vi "write initial config.vi"(8 "error in (no error)":errorcluster, 11 "Channel in":refnum<class "Channel.lvclass">) -> (0 "error out":errorcluster, 3 "Channel out":refnum<class "Channel.lvclass">)   [LabVIEW 2018, in "Channel.lvclass"]
uses:
  Channel.lvclass
  Channel.lvclass/Channel.ctl
  Simulated_CCD_Camera/Simulated Camera.lvclass
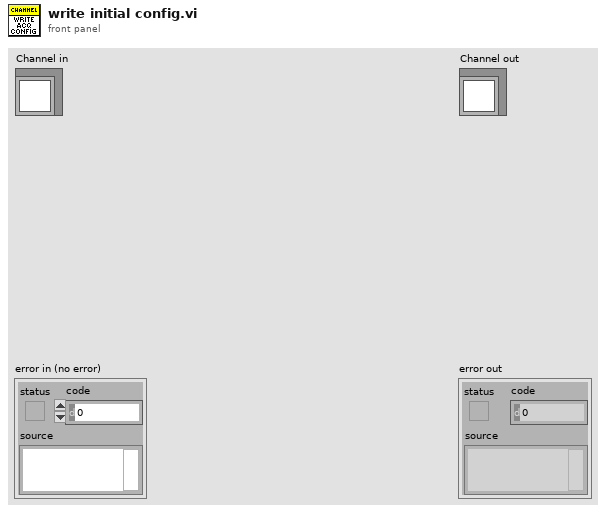
[diagram p1: front panel]
types:
  T1 = cluster{"EXPTIME":errorcluster, "#FRAMES":errorcluster, "#CYCLES":errorcluster, "WAVEPLATE_POS":errorcluster, "TEMP":errorcluster, "COOLER_POWER_STATUS":errorcluster, "SUFFIX":errorcluster}
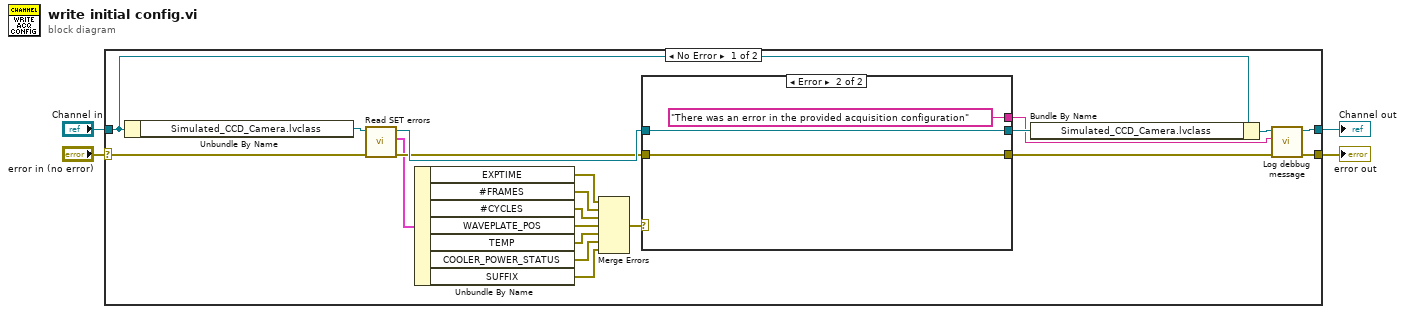
[diagram p0: block diagram]
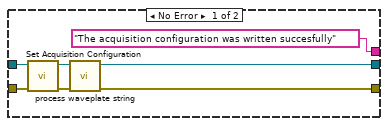
[diagram p2: hidden frame]
diagram:
  n1 = case shown="No Error" "error in (no error)" {
    selector: "error in (no error)" -> [w10 w36]
    tunnel: [w7 w36] -> w3
    tunnel: [w8 w35] -> w1
    tunnel: "Channel in" -> [w11 w35]
    frame No Error {
      n2 = Unbundle By Name(w11) -> ("Simulated_CCD_Camera.lvclass"=w23:refnum<class "Simulated Camera.lvclass">)
      n3 = call-dynamic "Read SET errors.vi"("error in (no error)"=w10, "Simulated Camera in"=w23) -> ("error out"=w21:errorcluster, "SET errors"=w20:T1, "Simulated Camera out"=w22:refnum<class "Simulated Camera.lvclass">)  [unwired: 7 in]
      n4 = Unbundle By Name(w20) -> ("EXPTIME"=w19:errorcluster, "#FRAMES"=w18:errorcluster, "#CYCLES"=w17:errorcluster, "WAVEPLATE_POS"=w16:errorcluster, "TEMP"=w15:errorcluster, "COOLER_POWER_STATUS"=w14:errorcluster, "SUFFIX"=w13:errorcluster)
      n5 = Merge Errors(w19, w18, w17, w16, w15, w14, w13) -> (w12:errorcluster)
      n6 = case shown="Error" w12 {
        tunnel: w22 -> [w30 w34]
        tunnel: w21 -> [w31 w33]
        tunnel: [w29 w33] -> w6
        tunnel: [w28 w34] -> w24
        tunnel: ["The acquisition configuration was written succesfully" ("String") "There was an error in the provided acquisition configuration" ("String")] -> w5
        frame No Error {
          n7 = call-dynamic "Set Acquisition Configuration.vi"("error in (no error)"=w31, "CCDCamera in"=w30) -> ("error out"=w26:errorcluster, "CCDCamera out"=w27:refnum<class "Simulated Camera.lvclass">)  [unwired: 8 in]
          n8 = call "process waveplate string.vi"("error in (no error)"=w26, "Simulated_CCD_Camera in"=w27) -> ("error out"=w29:errorcluster, "Simulated_CCD_Camera out"=w28:refnum<class "Simulated Camera.lvclass">)  [unwired: 8 in]
        }
        frame Error {
        }
      }
      n9 = Bundle By Name(cluster=w11, "Simulated_CCD_Camera.lvclass"=w24) -> (w9:refnum<class "Channel.lvclass">)
      n10 = call "Log debbug message.vi"("error in (no error)"=w6, "String"=w5, "Channel in"=w9) -> ("error out"=w7:errorcluster, "Channel out"=w8:refnum<class "Channel.lvclass">)  [unwired: 7 in]
    }
    frame Error {
    }
  }
  "error out" <- w3
  "Channel out" <- w1
